vi "Icai 105 - Simultry.vi"() -> ()   [LabVIEW 2010]
uses:
  <vilib>/Utility/error.llb/DialogType.ctl
  <vilib>/DAQmx/write.llb/DAQmx Write (Analog DBL 1Chan 1Samp).vi
  <vilib>/DAQmx/write.llb/DAQmx Write (Analog Wfm 1Chan NSamp).vi
  <vilib>/DAQmx/create/channels.llb/DAQmx Create Channel (AO-Voltage-Basic).vi
  <vilib>/daqmx/miscellaneous.llb/DAQmx Fill In Error Info.vi
  <vilib>/Waveform/WDTOps.llb/WDT Append Waveforms DBL.vi
  <vilib>/measure/NI_MABase.lvlib
  Program Files/National Instruments/LabVIEW 2010/resource/objmgr/daqmx.rc
panel:
  out "Name":refnum<k21>
  out "number of samples written per channel":u32
  out "max value":dbl
  in  "Logic Output Channel":tag="Dev1/ao3"
  in  "FM Waveform Channel":tag="Dev1/ao2"
  out "error out":errorcluster caption="error out (DAQ)"
  out "Mod":dbl=118572.0
  out "Numeric 2":dbl=3900000.0 format="%#_7g"
  out "Numeric":dbl=3900000.0 format="%#_7g"
  in  "CAI/ICAI":bool=TRUE
  in  "DC 2":ext=1140.74 format="%.2f"
  out "?":dbl=579698.7113293351 format="%#_6f"
  in  "Fs":dbl=1000000.0
  out "#s":dbl=39524.02451426849
  in  "Time int":i32=7200
  in  "Sensitivity":u16(ring)=21 items=["2 nV/fA", "5 nV/fA", "10 nV/fA", "20 nV/fA", "50 nV/fA", "100 nV/fA", "200 nV/fA", "500 nV/fA", "1 uV/pA", "2 uV/pA", "5 uV/pA", "10 uV/pA", "20 uV/pA", "50 uV/pA", "100 uV/pA", "200 uV/pA", "500 uV/pA", "1 mV/nA", "2 mV/nA", "5 mV/nA", "10 mV/nA", "20 mV/nA", "50 mV/nA", "100 mV/nA", "200 mV/nA", "500 mV/nA", "1 V/uA"]
  in  "Detection Bandwidth":u16(ring)=7 items=["25 kHz", "8.33 kHz", "2.50 kHz", "833 Hz", "250 Hz", "83.3 Hz", "25 Hz", "8.33 Hz", "2.50 Hz", "0.833 Hz", "0.250 Hz", "0.0833 Hz", "0.025 Hz"]
  in  "SR 830 GPIB Address":i32=8
  in  "Freq 2":dbl=2290.0 format="%_7g"
  out "Iterat #":dbl=10.0
  in  "Iteration":dbl=2.0
  in  "stop 2":bool
  in  "pulse":bool=TRUE
  in  "Start":ext=0.2
  out "?":waveform(dbl)[](graph)=[{"t0"=timestamp(0 s since 1904-01-01), "dt"=1e-06, "Y"=array[3900000 elements]}, {"t0"=timestamp(0 s since 1904-01-01), "dt"=1e-06, "Y"=array[3900000 elements]}]
  in  "amplitude 2":dbl=1.0 format="%0.2p"
  in  "?":T1(ring)=enum."Triangle Wave"
  in  "phase 2":dbl format="%.2p"
  in  "Offset 2":dbl=-0.0 format="%#_6p"
  in  "frequency 4":dbl=100.0 format="%0.2p"
  in  "sampling info 4":cluster{"Fs":dbl, "#s":dbl}={"Fs"=1000000.0, "#s"=2500.0} {"Fs" format="%.2p"}
  in  "?":T1(ring)=enum."Triangle Wave"
  in  "offset 4":dbl=-1.0 format="%0.2p"
  in  "phase 4":dbl=90.0 format="%.2p"
  in  "amplitude 4":dbl=1.0 format="%0.2p"
  in  "frequency 1":dbl=100.0 format="%0.2p"
  in  "amplitude 1":dbl=1.0 format="%0.2p"
  in  "sampling info 1":cluster{"Fs":dbl, "#s":dbl}={"Fs"=1000000.0, "#s"=2500.0} {"Fs" format="%.2p"}
  in  "?":T1(ring)=enum."Triangle Wave"
  in  "phase 1":dbl=-90.0 format="%.2p"
  in  "Offset 1":dbl format="%#_6p"
  in  "iterat":dbl=1.0
  out "CW":dbl=123571.0
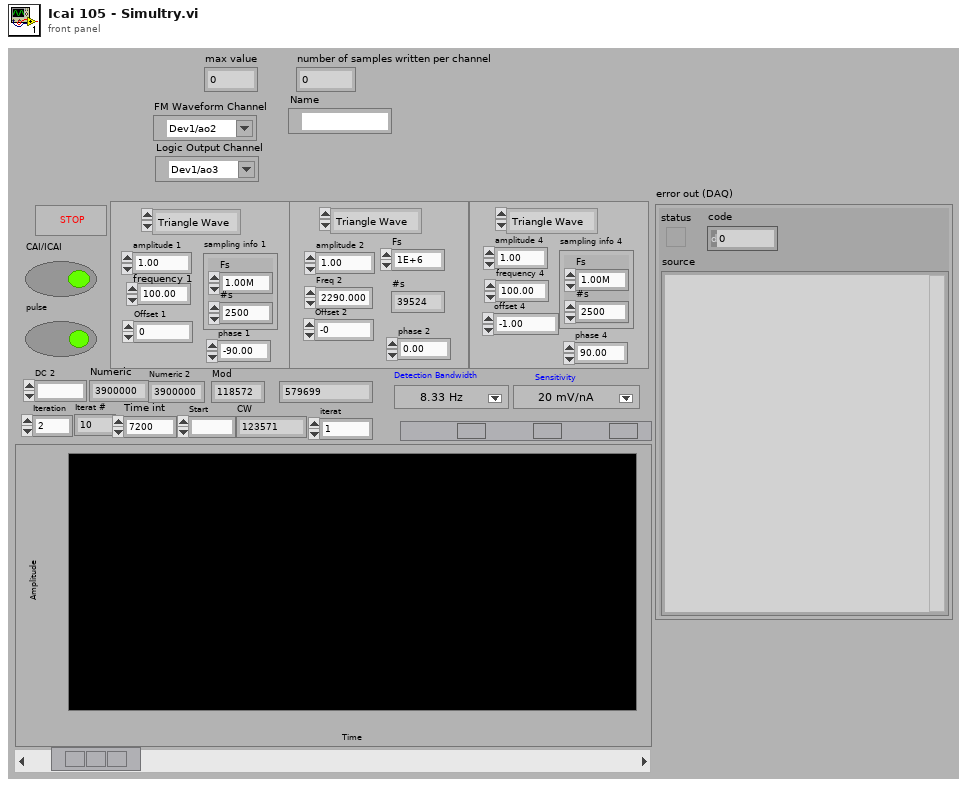
[diagram p1: front panel]
types:
  T1 = enum16{"Sine Wave", "Triangle Wave", "Square Wave", "Sawtooth Wave"}
  T2 = typedef "DialogType.ctl" = u16
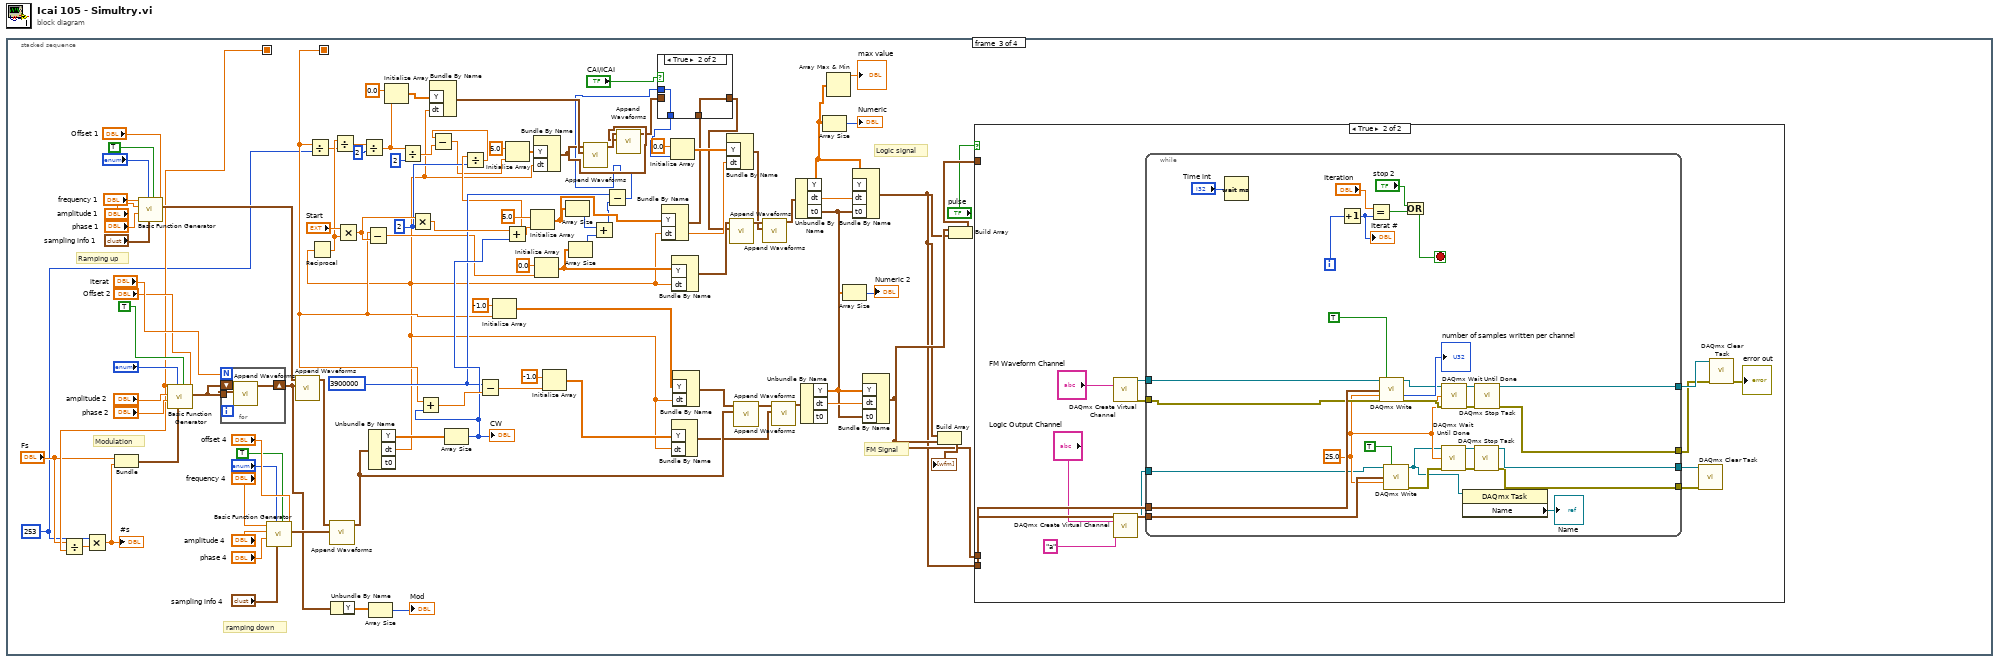
[diagram p0: block diagram]
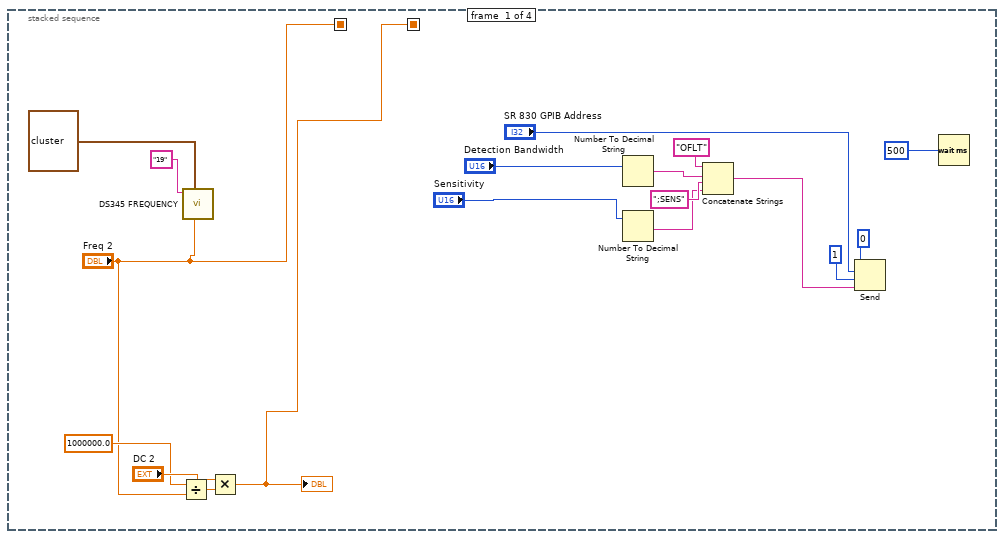
[diagram p2: hidden frame]
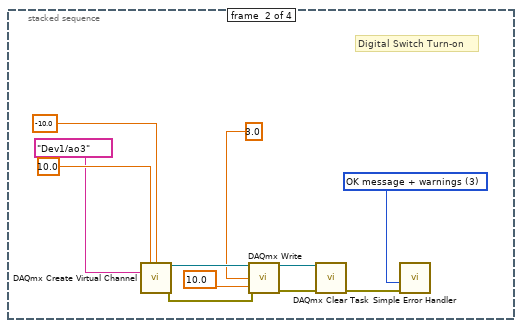
[diagram p3: hidden frame]
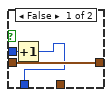
[diagram p4: hidden frame]
diagram:
  n1 = stacked-sequence {
    seq-local: ["Freq 2" _ _ _] -> [_ _ w71 _]
    seq-local: [w2 _ _ _] -> [_ _ w56 _]
    frame #0 {
      n2 = Divide(x=1000000.0 ("Fs 2"), y="Freq 2") -> (x/y=w5:dbl)
      n3 = call "DS345 FREQUENCY.vi"("GPIB address"="19", "amplitude (0 Vrms:0)"=cluster{ext, i32} {0.02, 0} ("Driving amplitude (0 Vrms:0)"), "frequency"="Freq 2") -> ()  [unwired: 5 in, 1 out]
      n4 = Multiply(x="DC 2", y=w5) -> (x*y=w2:ext)
      "?" <- w2
      n5 = Number To Decimal String(number="Detection Bandwidth") -> (decimal integer string=w15:string)  [unwired: 1 out]
      n6 = Number To Decimal String(number="Sensitivity") -> (decimal integer string=w13:string)  [unwired: 1 out]
      n7 = Concatenate Strings("OFLT", w15, ";SENS", w13) -> (w12:string)
      n8 = Send(0:0 ("bus"), 2:"SR 830 GPIB Address", 3:i16 1 ("mode"), 5:w12) -> ()  [unwired: 1 in, 3 out]
      n9 = Wait (ms)(milliseconds to wait=500) -> ()  [unwired: 1 out]
    }
    frame #1 {
      w22 = T2 3 items=["no dialog", "OK message", "continue or stop message", "OK message + warnings", "continue/stop + warnings"] ("type of dialog (OK msg:1)")
      # "Digital Switch Turn-on"
      n10 = call-poly <vilib>:"DAQmx Create Virtual Channel.vi"("maximum value"=10.0 ("Maximum Value"), "minimum value"=-10.0 ("Minimum Value"), "physical channels"=tag "Dev1/ao3" ("Physical Channel")) -> ("task out"=w25:refnum<k21>, "error out"=w26:errorcluster)  [unwired: 6 in, 5 out]
      n11 = call-poly <vilib>:"DAQmx Write.vi"("task/channels in"=w25, "data"=3.0 ("Voltage Output"), "timeout"=10.0, "error in"=w26) -> ("task out"=w20:refnum<k21>, "error out"=w21:errorcluster)  [unwired: 1 in, 9 out]
      n12 = call <vilib>:"DAQmx Clear Task.vi"("task in"=w20, "error in"=w21) -> ("error out"=w19:errorcluster)  [unwired: 13 out]
      n13 = call <vilib>:"Simple Error Handler.vi"("type of dialog (OK msg:1)"=w22, "error in (no error)"=w19) -> ()  [unwired: 8 out]
    }
    frame #2 {
      w48 = 253
      w64 = 2
      w89 = 3900000
      # "FM Signal"
      # "Logic signal"
      # "Ramping up"
      # "ramping down"
      # "Modulation"
      n14 = Divide(x="Fs", y=w71) -> (x/y=w70:dbl)
      n15 = Multiply(x=w48, y=w70) -> (x*y=w68:dbl)
      "#s" <- w68
      n16 = Bundle("Fs"="Fs", w68) -> (w67:cluster{"Fs":dbl, dbl})  [unwired: 1 out]
      n17 = call <vilib>:"Basic Function Generator.vi"("offset"="Offset 1", "reset signal"=TRUE, "sampling info"="sampling info 1", "signal type"="?", "phase"="phase 1", "amplitude"="amplitude 1", "frequency"="frequency 1") -> ("signal out"=w111:waveform(dbl))  [unwired: 2 in, 2 out]
      n18 = call <vilib>:"Basic Function Generator.vi"("offset"="Offset 2", "reset signal"=TRUE, "sampling info"=w67, "signal type"="?", "phase"="phase 2", "amplitude"="amplitude 2", "frequency"=w71) -> ("signal out"=w72:waveform(dbl))  [unwired: 2 in, 2 out]
      n19 = for {
        N: "iterat" -> [_]
        shift-right: [w182] -> w34
        shift-left: w72 -> [w180]
        tunnel: w72 -> [w181]
        n20 = call-poly <vilib>:"Append Waveforms.vi"("waveform B"=w181, "waveform A"=w180) -> ("waveform out"=w182:waveform(dbl))  [unwired: 1 in, 8 out]
      }
      n21 = call <vilib>:"Basic Function Generator.vi"("offset"="offset 4", "reset signal"=TRUE, "sampling info"="sampling info 4", "signal type"="?", "phase"="phase 4", "amplitude"="amplitude 4", "frequency"="frequency 4") -> ("signal out"=w116:waveform(dbl))  [unwired: 2 in, 2 out]
      n22 = call-poly <vilib>:"Append Waveforms.vi"("waveform B"=w34, "waveform A"=w111) -> ("waveform out"=w110:waveform(dbl))  [unwired: 1 in, 8 out]
      n23 = Divide(x=w56, y=w48) -> (x/y=w57:ext)
      n24 = call-poly <vilib>:"Append Waveforms.vi"("waveform B"=w116, "waveform A"=w110) -> ("waveform out"=w109:waveform(dbl))  [unwired: 1 in, 8 out]
      n25 = Unbundle By Name(w34) -> ("Y"=w35:dbl[])
      n26 = Array Size(array=w35) -> (size(s)=→"Mod":i32)
      n27 = Unbundle By Name(w109) -> ("Y"=w112:dbl[], "dt"=w47:dbl)  [unwired: 1 out]
      n28 = Reciprocal(x=w47) -> (1/x=w58:dbl)
      n29 = Divide(x=w58, y=w57) -> (x/y=w54:ext)
      n30 = Multiply(x="Start", y=w58) -> (x*y=w83:ext)
      n31 = Divide(x=w54, y=2) -> (x/y=w51:ext)
      n32 = Subtract(x=w56, y=w83) -> (x-y=w84:ext)
      n33 = Initialize Array(0.0 ("Trigger down"), w51) -> (w61:dbl[])
      n34 = Divide(x=w51, y=2) -> (x/y=w49:ext)
      n35 = Multiply(x=w83, y=w64) -> (x*y=w91:ext)
      n36 = Bundle By Name("Y"=w61, "dt"=w47) -> (w60:waveform(dbl))  [unwired: 1 out]
      n37 = Array Size(array=w112) -> (size(s)=w90:i32)
      "CW" <- w90
      n38 = Add(x=w56, y=w90) -> (x+y=w95:ext)
      n39 = Subtract(x=w89, y=w95) -> (x-y=w94:ext)
      n40 = Initialize Array(-1.0 ("DC level"), w56) -> (w97:dbl[])
      n41 = Add(x=w91, y=w90) -> (x+y=w65:ext)
      n42 = Divide(x=w65, y=w64) -> (x/y=w53:ext)
      n43 = Subtract(x=w53, y=w49) -> (x-y=w52:ext)
      n44 = Initialize Array(5.0 ("Trigger up"), w52) -> (w63:dbl[])
      n45 = Initialize Array(5.0 ("Trigger up"), w65) -> (w81:dbl[])
      n46 = Bundle By Name("Y"=w63, "dt"=w47) -> (w46:waveform(dbl))  [unwired: 1 out]
      n47 = Initialize Array(0.0 ("Trigger down"), w84) -> (w82:dbl[])
      n48 = Initialize Array(-1.0 ("DC level"), w94) -> (w93:dbl[])
      n49 = Array Size(array=w81) -> (size(s)=w79:i32)
      n50 = Array Size(array=w82) -> (size(s)=w80:i32)
      n51 = call-poly <vilib>:"Append Waveforms.vi"("waveform B"=w60, "waveform A"=w46) -> ("waveform out"=w59:waveform(dbl))  [unwired: 1 in, 8 out]
      n52 = Add(x=w79, y=w80) -> (x+y=w78:i32)
      n53 = Subtract(x=w89, y=w78) -> (x-y=w38:i32)
      n54 = call-poly <vilib>:"Append Waveforms.vi"("waveform B"=w46, "waveform A"=w59) -> ("waveform out"=w45:waveform(dbl))  [unwired: 1 in, 8 out]
      n55 = Bundle By Name("Y"=w81, "dt"=w47) -> (w43:waveform(dbl))  [unwired: 1 out]
      n56 = case shown="True" "CAI/ICAI" {
        tunnel: w45 -> [w135 _]
        tunnel: [w135 w137] -> w44
        tunnel: w43 -> [_ w137]
        tunnel: w38 -> [w134 w136]
        tunnel: [w133 w136] -> w37
        frame False {
          n57 = Increment(x=w134) -> (x+1=w133:i32)
        }
        frame True {
        }
      }
      n58 = Initialize Array(0.0 ("Trigger down"), w37) -> (w87:dbl[])
      n59 = Bundle By Name("Y"=w93, "dt"=w47) -> (w92:waveform(dbl))  [unwired: 1 out]
      n60 = Bundle By Name("Y"=w82, "dt"=w47) -> (w86:waveform(dbl))  [unwired: 1 out]
      n61 = Bundle By Name("Y"=w97, "dt"=w47) -> (w114:waveform(dbl))  [unwired: 1 out]
      n62 = Bundle By Name("Y"=w87, "dt"=w47) -> (w85:waveform(dbl))  [unwired: 1 out]
      n63 = call-poly <vilib>:"Append Waveforms.vi"("waveform B"=w44, "waveform A"=w86) -> ("waveform out"=w106:waveform(dbl))  [unwired: 1 in, 8 out]
      n64 = call-poly <vilib>:"Append Waveforms.vi"("waveform B"=w109, "waveform A"=w114) -> ("waveform out"=w115:waveform(dbl))  [unwired: 1 in, 8 out]
      n65 = call-poly <vilib>:"Append Waveforms.vi"("waveform B"=w85, "waveform A"=w106) -> ("waveform out"=w102:waveform(dbl))  [unwired: 1 in, 8 out]
      n66 = call-poly <vilib>:"Append Waveforms.vi"("waveform B"=w92, "waveform A"=w115) -> ("waveform out"=w100:waveform(dbl))  [unwired: 1 in, 8 out]
      n67 = Unbundle By Name(w102) -> ("Y"=w33:dbl[], "dt"=w101:dbl, "t0"=w77:timestamp)
      n68 = Unbundle By Name(w100) -> ("Y"=w39:dbl[], "dt"=w99:dbl)  [unwired: 1 out]
      n69 = Array Size(array=w33) -> (size(s)=→"Numeric":i32)
      n70 = Array Max & Min(array=w33) -> (max value=→"max value":dbl)  [unwired: 3 out]
      n71 = Array Size(array=w39) -> (size(s)=→"Numeric 2":i32)
      n72 = Bundle By Name("Y"=w33, "dt"=w101, "t0"=w77) -> (w30:waveform(dbl))  [unwired: 1 out]
      n73 = Bundle By Name("Y"=w39, "dt"=w99, "t0"=w77) -> (w31:waveform(dbl))  [unwired: 1 out]
      n74 = Build Array(w30, w31) -> (→"?":waveform(dbl)[])
      n75 = Build Array(w31, w30) -> (w103:waveform(dbl)[])
      n76 = case shown="True" "pulse" {
        tunnel: w103 -> [_ _]
        tunnel: w31 -> [_ w150]
        tunnel: w30 -> [_ w146]
        frame False {
        }
        frame True {
          n77 = call-poly <vilib>:"DAQmx Create Virtual Channel.vi"("physical channels"="FM Waveform Channel") -> ("task out"=w148:refnum<k21>, "error out"=w147:errorcluster)  [unwired: 13 in]
          n78 = call-poly <vilib>:"DAQmx Create Virtual Channel.vi"("physical channels"="Logic Output Channel", "name to assign"="a") -> ("task out"=w144:refnum<k21>)  [unwired: 12 in, 1 out]
          n79 = while {
            tunnel: w150 -> [w166]
            tunnel: w148 -> [w160]
            tunnel: w147 -> [w159]
            tunnel: w146 -> [w163]
            tunnel: w144 -> [w157]
            tunnel: [w154] -> w142
            tunnel: [w153] -> w141
            tunnel: [w152] -> w140
            tunnel: [w151] -> w139
            i -> [w176]
            stop <- w177 stop-if-true
            w158 = 25.0 ("timeout (s)")
            n80 = Wait (ms)(milliseconds to wait="Time int") -> ()  [unwired: 1 out]
            n81 = Increment(x=w176) -> (x+1=w174:i32)
            "Iterat #" <- w174
            n82 = Equal?(x="Iteration", y=w174) -> (x = y?=w179:bool)
            n83 = call-poly <vilib>:"DAQmx Write.vi"("task/channels in"=w160, "auto start"=TRUE, "data"=w166, "timeout"=w158, "error in"=w159) -> ("task out"=w168:refnum<k21>, "number of samples written per channel"=→"number of samples written per channel":u32, "error out"=w167:errorcluster)  [unwired: 8 in]
            n84 = call-poly <vilib>:"DAQmx Write.vi"("task/channels in"=w157, "auto start"=TRUE, "data"=w163, "timeout"=w158) -> ("task out"=w156:refnum<k21>, "error out"=w164:errorcluster)  [unwired: 9 in, 1 out]
            n85 = Or(x="stop 2", y=w179) -> (x .or. y?=w177:bool)
            n86 = call <vilib>:"DAQmx Wait Until Done.vi"("task/channels in"=w156, "timeout (sec)"=w158, "error in"=w164) -> ("task out"=w162:refnum<k21>, "error out"=w165:errorcluster)  [unwired: 11 in]
            n87 = call <vilib>:"DAQmx Wait Until Done.vi"("task/channels in"=w168, "timeout (sec)"=w158, "error in"=w167) -> ("task out"=w172:refnum<k21>, "error out"=w171:errorcluster)  [unwired: 11 in]
            n88 = property class="DAQmx Task"(reference=w156) -> ("Name"=→"Name":refnum<k21>)  [unwired: 1 in, 2 out]
            n89 = call <vilib>:"DAQmx Stop Task.vi"("task/channels in"=w162, "error in"=w165) -> ("task out"=w154:refnum<k21>, "error out"=w153:errorcluster)  [unwired: 12 in]
            n90 = call <vilib>:"DAQmx Stop Task.vi"("task/channels in"=w172, "error in"=w171) -> ("task out"=w152:refnum<k21>, "error out"=w151:errorcluster)  [unwired: 12 in]
          }
          n91 = call <vilib>:"DAQmx Clear Task.vi"("task in"=w142, "error in"=w141) -> ()  [unwired: 13 in, 1 out]
          n92 = call <vilib>:"DAQmx Clear Task.vi"("task in"=w140, "error in"=w139) -> ("error out"=→"error out":errorcluster)  [unwired: 13 in]
        }
      }
    }
    frame #3 {
    }
  }
